vi "시리얼 통신 문자열 변환 실습.vi"() -> ()   [LabVIEW 2020]
panel:
  in  "숫자형":i32=1
  out "연결된 문자열":string
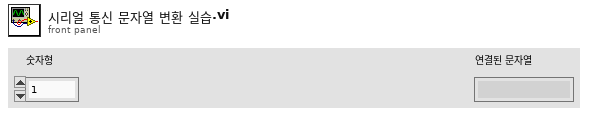
[diagram p1: front panel]
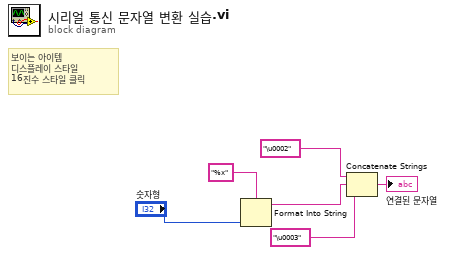
[diagram p0: block diagram]
diagram:
  # "보이는 아이템\n디스플레이 스타일\n16진수 스타일 클릭"
  n1 = Format Into String(format string="%x" ("포맷 문자열"), "숫자형") -> (resulting string=w3:string)  [unwired: 2 in, 1 out]
  n2 = Concatenate Strings("\u0002", w3, "\u0003") -> (→"연결된 문자열":string)
